vi "Associate a File Extension.vi"(8 "error in (no error)":errorcluster, 10 "string":string=".myext", 11 "exe path":path) -> (0 "error out":errorcluster, 3 "exe path (dup)":path)   [LabVIEW 2014]
uses:
  <vilib>/registry/registry.llb/Registry RtKey.ctl
  <vilib>/registry/registry.llb/Write Registry Value Simple STR.vi
panel:
  out "concatenated string 2":string
  out "concatenated string":string
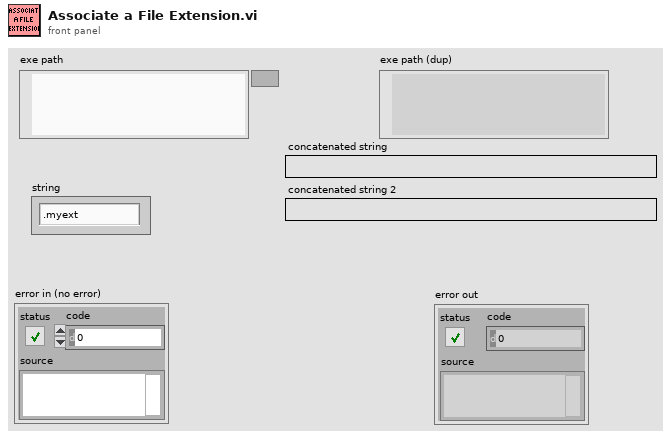
[diagram p1: front panel]
types:
  T1 = typedef "Registry RtKey.ctl" = enum32{"HKEY_CLASSES_ROOT", "HKEY_CURRENT_USER", "HKEY_LOCAL_MACHINE", "HKEY_USERS", "HKEY_PERFORMANCE_DATA", "HKEY_CURRENT_CONFIG", "HKEY_DYN_DATA"}
  T2 = typedef "Registry refnum.ctl" = refnum<k1>
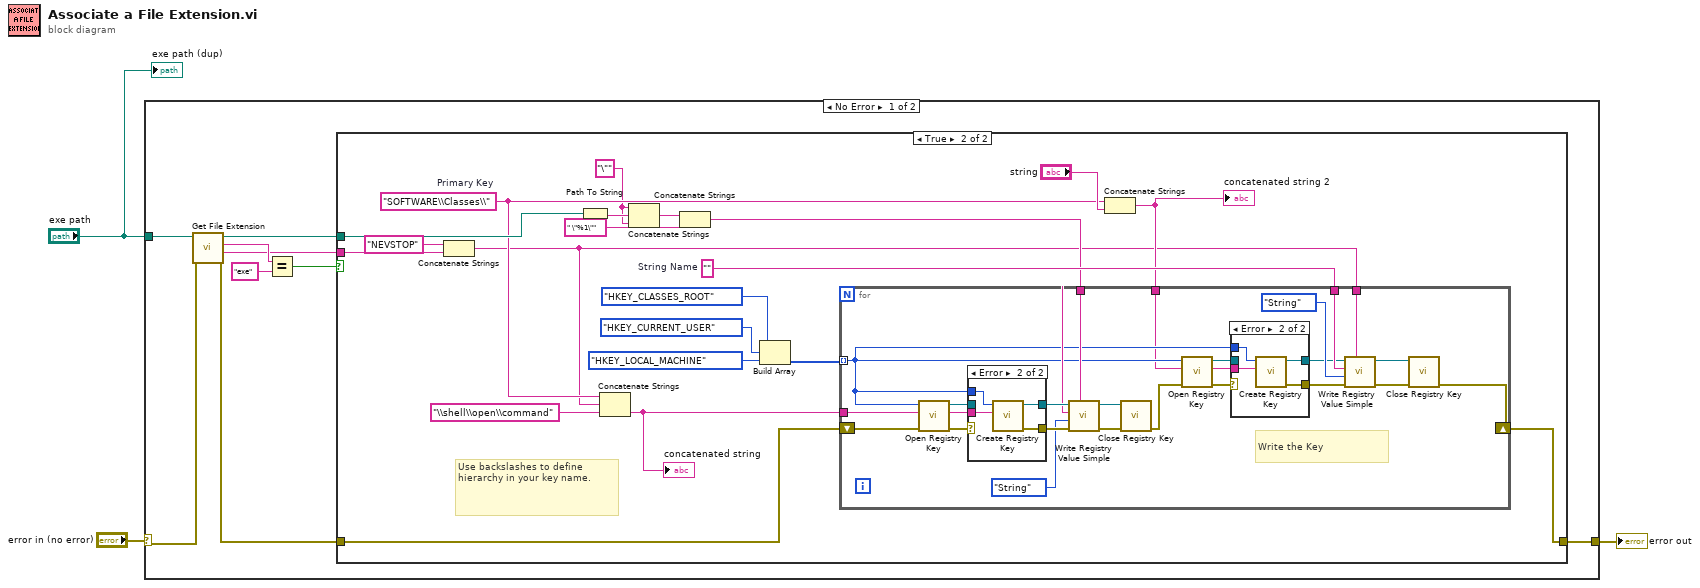
[diagram p0: block diagram]
diagram:
  n1 = case shown="No Error" "error in (no error)" {
    selector: "error in (no error)" -> [w8 w70]
    tunnel: [w12 w70] -> w3
    tunnel: "exe path" -> [w11 _]
    frame No Error {
      n2 = call <vilib>:"Get File Extension.vi"("error in (no error)"=w8, "file"=w11) -> ("error out"=w7:errorcluster, "filename without extension"=w4:string, "lowercase file extension"=w5:string, "dup file"=w6:path)  [unwired: 6 in]
      n3 = Equal?(x=w5, y="exe") -> (x = y?=w9:bool)
      n4 = case shown="True" w9 {
        tunnel: [w13 w33] -> w12
        tunnel: w7 -> [w13 w25]
        tunnel: w4 -> [_ w23]
        tunnel: w6 -> [_ w31]
        frame False {
        }
        frame True {
          w17 = "\"" ("string")
          w21 = "SOFTWARE\\Classes\\"  # Primary Key
          w32 = ""  # String Name
          # "Use backslashes to define hierarchy in your key name."
          n5 = Concatenate Strings("NEVSTOP" ("string"), w23) -> (w20:string)
          n6 = Path To String(path=w31) -> (string=w30:string)
          n7 = Concatenate Strings(w21, w20, "\\shell\\open\\command" ("subkey")) -> (w26:string)
          "concatenated string" <- w26
          n8 = Concatenate Strings(w17, w30, w17) -> (w18:string)
          n9 = Concatenate Strings(w18, " \"%1\"" ("string")) -> (w28:string)
          n10 = Build Array(Registry_RtKey."HKEY_CLASSES_ROOT" ("Root Key"), Registry_RtKey."HKEY_CURRENT_USER" ("Root Key"), Registry_RtKey."HKEY_LOCAL_MACHINE" ("Root Key")) -> (w16:T1[])
          n11 = Concatenate Strings(w21, "string") -> (w22:string)
          "concatenated string 2" <- w22
          n12 = for {
            tunnel: w32 -> [w48]
            tunnel: w28 -> [w47]
            tunnel: w26 -> [w46]
            tunnel: w16 -> [w38] mode=indexing
            tunnel: w22 -> [w36]
            tunnel: w20 -> [w35]
            shift-right: [w49] -> w33
            shift-left: w25 -> [w45]
            # "Write the Key"
            n13 = call <vilib>:"Open Registry Key.vi"("error in (no error)"=w45, "subkey"=w46, "root key (HKEY_LOCAL_MACHINE)"=w38) -> ("error out"=w44:errorcluster, "refnum out"=w43:T2)  [unwired: 7 in]
            n14 = case shown="Error" w44 {
              selector: w44 -> [w65 _]
              tunnel: [w65 w69] -> w57
              tunnel: [w64 w68] -> w55
              tunnel: w38 -> [_ w67]
              tunnel: w46 -> [_ w66]
              tunnel: w43 -> [w64 _]
              frame No Error {
              }
              frame Error {
                n15 = call <vilib>:"Create Registry Key.vi"("subkey"=w66, "root key (HKEY_LOCAL_MACHINE)"=w67) -> ("error out"=w69:errorcluster, "refnum out"=w68:T2)  [unwired: 7 in, 1 out]
              }
            }
            n16 = call-poly <vilib>:"Write Registry Value Simple.vi"("String/Binary data"=w47, "error in (no error)"=w57, "simple data type"=enum16{"String", "Binary", "DWORD"}."String", "value"=w48, "refnum"=w55) -> ("error out"=w53:errorcluster, "refnum out"=w54:T2)  [unwired: 3 in]
            n17 = call <vilib>:"Close Registry Key.vi"("error in (no error)"=w53, "refnum"=w54) -> ("error out"=w37:errorcluster)  [unwired: 5 in]
            n18 = call <vilib>:"Open Registry Key.vi"("error in (no error)"=w37, "subkey"=w36, "root key (HKEY_LOCAL_MACHINE)"=w38) -> ("error out"=w41:errorcluster, "refnum out"=w42:T2)  [unwired: 7 in]
            n19 = case shown="Error" w41 {
              selector: w41 -> [w59 _]
              tunnel: [w59 w63] -> w40
              tunnel: [w58 w62] -> w39
              tunnel: w38 -> [_ w61]
              tunnel: w36 -> [_ w60]
              tunnel: w42 -> [w58 _]
              frame No Error {
              }
              frame Error {
                n20 = call <vilib>:"Create Registry Key.vi"("subkey"=w60, "root key (HKEY_LOCAL_MACHINE)"=w61) -> ("error out"=w63:errorcluster, "refnum out"=w62:T2)  [unwired: 7 in, 1 out]
              }
            }
            n21 = call-poly <vilib>:"Write Registry Value Simple.vi"("String/Binary data"=w35, "error in (no error)"=w40, "simple data type"=enum16{"String", "Binary", "DWORD"}."String", "value"=w48, "refnum"=w39) -> ("error out"=w52:errorcluster, "refnum out"=w51:T2)  [unwired: 3 in]
            n22 = call <vilib>:"Close Registry Key.vi"("error in (no error)"=w52, "refnum"=w51) -> ("error out"=w49:errorcluster)  [unwired: 5 in]
          }
        }
      }
    }
    frame Error {
    }
  }
  "error out" <- w3
  "exe path (dup)" <- "exe path"
